vi "MH_CalcDeltaTNeg.vi"(5 "Buffsize":i32, 6 "WinIndex":i32, 7 "TrueTime":u64, 9 "WIndowW":i32, 10 "Data In":u64[](array[numeric]), 11 "Buffindex":i32) -> (1 "WinIndexOut":i32, 2 "NewDelta":bool, 3 "DeltaT Out":i32[](array[numeric]))   [LabVIEW 2019]
panel:
  # "here"
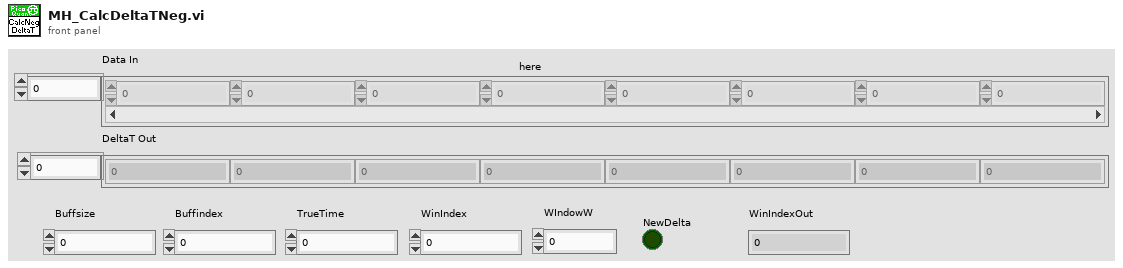
[diagram p1: front panel]
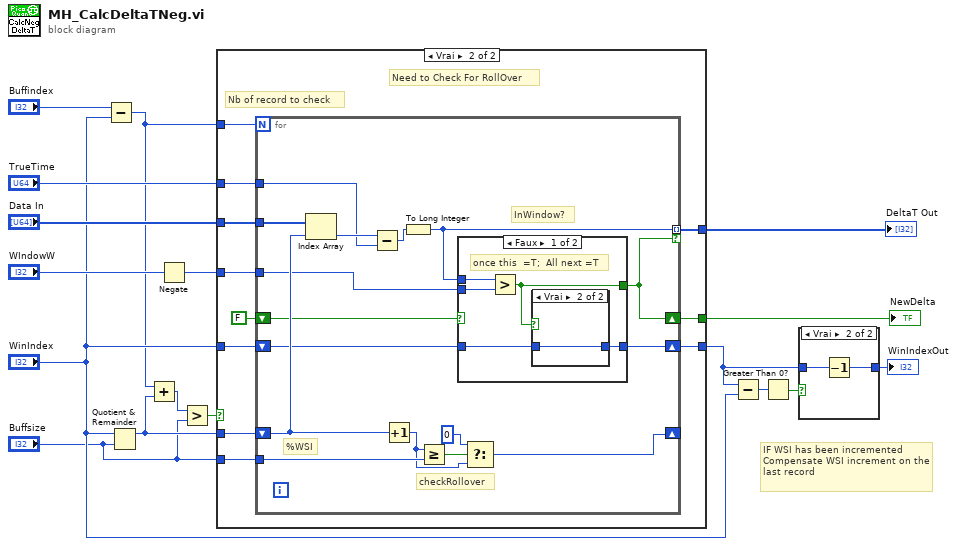
[diagram p0: block diagram]
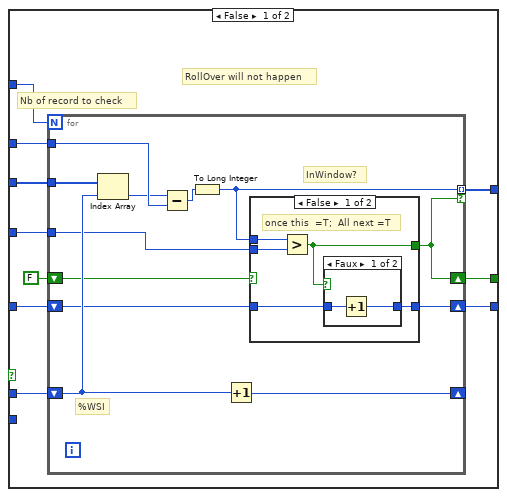
[diagram p2: hidden frame]
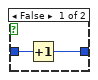
[diagram p5: hidden frame]
diagram:
  # "IF WSI has been incremented\nCompensate WSI increment on the last record"
  n1 = Subtract(x="Buffindex", y="WinIndex") -> (x-y=w6:i32)
  n2 = Quotient & Remainder(x="WinIndex", y="Buffsize") -> (x-y*floor(x/y)=w5:i32)  [unwired: 1 out]
  n3 = Add(x=w6, y=w5) -> (x+y=w4:i32)
  n4 = Negate(x="WIndowW") -> (-x=w1:i32)
  n5 = Greater?(x=w4, y="Buffsize") -> (0:w2:bool)
  n6 = case shown="Vrai" w2 {
    tunnel: "Data In" -> [w27 w60]
    tunnel: "TrueTime" -> [w26 w59]
    tunnel: w1 -> [w25 w58]
    tunnel: [w24 w57] -> w13
    tunnel: [w23 w56] -> w12
    tunnel: "WinIndex" -> [w21 w54]
    tunnel: [w20 w53] -> w7
    tunnel: w6 -> [w19 w52]
    tunnel: w5 -> [w18 w51]
    tunnel: "Buffsize" -> [_ w50]
    frame False {
      # "RollOver will not happen"
      # "Nb of record to check"
      n7 = for {
        N: w19 -> [_]
        tunnel: w27 -> [w39]
        tunnel: w26 -> [w30]
        tunnel: [w28] -> w24 mode=indexing if=w35
        shift-right: [w32] -> w20
        shift-left: w21 -> [w33]
        shift-right: [w31] -> _
        shift-left: w18 -> [w37]
        tunnel: w25 -> [w36]
        shift-right: [w35] -> w23
        shift-left: FALSE -> [w34]
        # "InWindow?"
        # "%WSI"
        n8 = Index Array(array=w39, index=w37) -> (element=w29:u64)
        n9 = Subtract(x=w29, y=w30) -> (x-y=w38:u64)
        n10 = To Long Integer(number=w38) -> (32bit integer=w28:i32)
        n11 = Increment(x=w37) -> (x+1=w31:i32)
        n12 = case shown="Vrai" w34 {
          selector: w34 -> [_ w48]
          tunnel: w28 -> [w44 _]
          tunnel: w36 -> [w43 _]
          tunnel: [w40 w48] -> w35
          tunnel: w33 -> [w42 w49]
          tunnel: [w41 w49] -> w32
          frame False {
            # "once this  =T;  All next =T"
            n13 = Greater?(x=w44, y=w43) -> (0:w40:bool)
            n14 = case shown="Faux" w40 {
              tunnel: w42 -> [w46 w47]
              tunnel: [w45 w47] -> w41
              frame False {
                n15 = Increment(x=w46) -> (x+1=w45:i32)
              }
              frame True {
              }
            }
          }
          frame True {
          }
        }
      }
    }
    frame True {
      # "Need to Check For RollOver"
      # "Nb of record to check"
      n16 = for {
        N: w52 -> [_]
        tunnel: w60 -> [w76]
        tunnel: w59 -> [w63]
        tunnel: [w61] -> w57 mode=indexing if=w71
        shift-right: [w68] -> w53
        shift-left: w54 -> [w69]
        shift-right: [w73] -> _
        shift-left: w51 -> [w74]
        tunnel: w50 -> [w75]
        tunnel: w58 -> [w72]
        shift-right: [w71] -> w56
        shift-left: FALSE -> [w70]
        # "checkRollover"
        # "InWindow?"
        # "%WSI"
        n17 = Index Array(array=w76, index=w74) -> (element=w64:u64)
        n18 = Subtract(x=w64, y=w63) -> (x-y=w62:u64)
        n19 = Increment(x=w74) -> (x+1=w65:i32)
        n20 = To Long Integer(number=w62) -> (32bit integer=w61:i32)
        n21 = Greater Or Equal?(x=w65, y=w75) -> (x >= y?=w67:bool)
        n22 = case shown="Faux" w70 {
          selector: w70 -> [_ w85]
          tunnel: w61 -> [w81 _]
          tunnel: w72 -> [w80 _]
          tunnel: [w77 w85] -> w71
          tunnel: w69 -> [w79 w86]
          tunnel: [w78 w86] -> w68
          frame False {
            # "once this  =T;  All next =T"
            n23 = Greater?(x=w81, y=w80) -> (0:w77:bool)
            n24 = case shown="Vrai" w77 {
              tunnel: w79 -> [w83 w84]
              tunnel: [w82 w84] -> w78
              frame False {
                n25 = Increment(x=w83) -> (x+1=w82:i32)
              }
              frame True {
              }
            }
          }
          frame True {
          }
        }
        n26 = Select(t=0 ("x+1"), s=w67, f=w65) -> (s? t:f=w73:i32)
      }
    }
  }
  "DeltaT Out" <- w13
  "NewDelta" <- w12
  n27 = Subtract(x=w7, y="WinIndex") -> (x-y=w10:i32)
  n28 = Greater Than 0?(x=w10) -> (x > 0?=w9:bool)
  n29 = case shown="Vrai" w9 {
    tunnel: [w87 w88] -> w8
    tunnel: w7 -> [w87 w89]
    frame False {
    }
    frame True {
      n30 = Decrement(x=w89) -> (x-1=w88:i32)
    }
  }
  "WinIndexOut" <- w8
